vi "LVClass_Camera set nbImagesToSum.vi"(0 "Camera in":refnum<class "Camera.lvclass">, 5 "nb_image":u32, 11 "error in (no error)":errorcluster) -> (4 "Camera out":refnum<class "Camera.lvclass">, 15 "error out":errorcluster)   [LabVIEW 2020, in "Camera.lvclass"]
doc: "Set number of images to sum.\n\n--------------------------------------------------------------------------------\n\n<B>CameraIn </B> : Camera object.\n<B>CameraOut </B> : Camera object.\n<B>images_count </B> : Images count.\n<B>ErrorIn </B> : Error\n<B>ErrorOut </B> : Error\n\n--------------------------------------------------------------------------------"
uses:
  Camera.lvclass
  Camera.lvclass/Camera.ctl
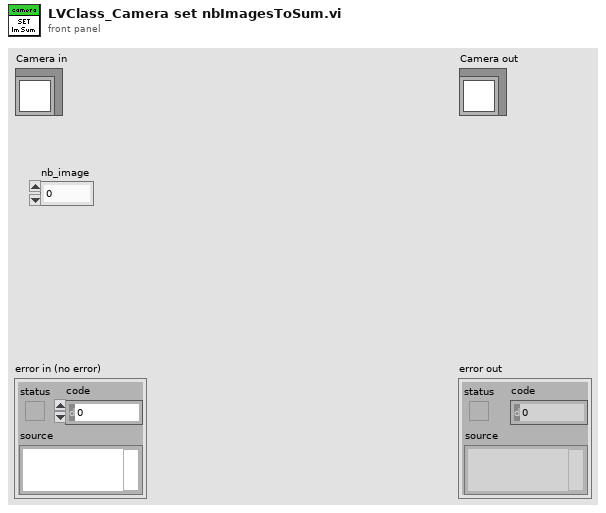
[diagram p1: front panel]
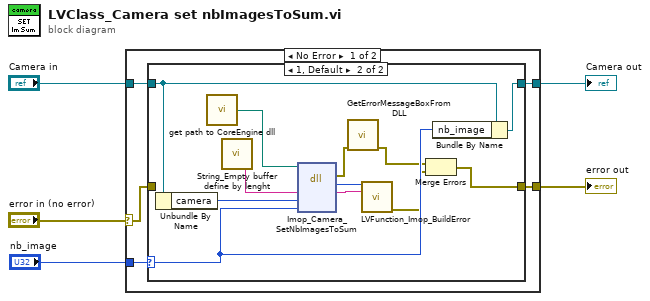
[diagram p0: block diagram]
diagram:
  n1 = case shown="No Error" "error in (no error)" {
    selector: "error in (no error)" -> [w6 w26]
    tunnel: [w10 w26] -> w4
    tunnel: [w8 w25] -> w2
    tunnel: "Camera in" -> [w9 w25]
    tunnel: "nb_image" -> [w7 _]
    frame No Error {
      n2 = case shown="1, Default" w7 {
        selector: w7 -> [_ w16]
        tunnel: [w11 w13] -> w10
        tunnel: w9 -> [w12 w18]
        tunnel: [w12 w17] -> w8
        tunnel: w6 -> [w11 _]
        frame 0 {
        }
        frame 1, Default {
          n3 = Unbundle By Name(w18) -> ("camera"=w21:i32)
          n4 = call "get path to CoreEngine dll.vi"() -> ("path to c_interface_vc100.dll"=w20:path)  [unwired: 12 in, 3 out]
          n5 = call "String_Empty buffer define by lenght.vi"() -> ("Empty buffer"=w24:string)  [unwired: 1 in]
          n6 = dll-call lib="D:/2_trunk/Soft_haso/ImOpCoreEngine4_LV2011/DLLs/ImopEngine4_vc100.dll" fn="Imop_Camera_SetNbImagesToSum"(path in=w20, "message"=w24, "camera"=w21, "nb_image"=w16) -> (error out=w19:errorcluster, "return type"=w23:i32, "message"=w22:string)  [unwired: 4 in, 1 out]
          n7 = call "GetErrorMessageBoxFromDLL.vi"("error IN"=w19) -> ("error OUT"=w15:errorcluster)  [unwired: 10 in]
          n8 = call "LVFunction_Imop_BuildError.vi"("code"=w23, "String to Prepend to source (\"\")"=w22) -> ("error out"=w14:errorcluster)  [unwired: 13 in]
          n9 = Merge Errors(w15, w14) -> (w13:errorcluster)
          n10 = Bundle By Name(cluster=w18, "nb_image"=w16) -> (w17:refnum<class "Camera.lvclass">)
        }
      }
    }
    frame Error {
    }
  }
  "error out" <- w4
  "Camera out" <- w2
